vi "cm2nm_createGraphEnteredPoints.vi"(1 "EnteredPoints_in":T1[](array[typedef])) -> (0 "XY_graphOut":cluster{dbl[], dbl[]}[](array[cluster]))   [LabVIEW 2011]
doc: "Create a graph of the points in a data set by group number. There will be a separate line for each group number."
uses:
  cm2nm_coordinate_information_v2.ctl
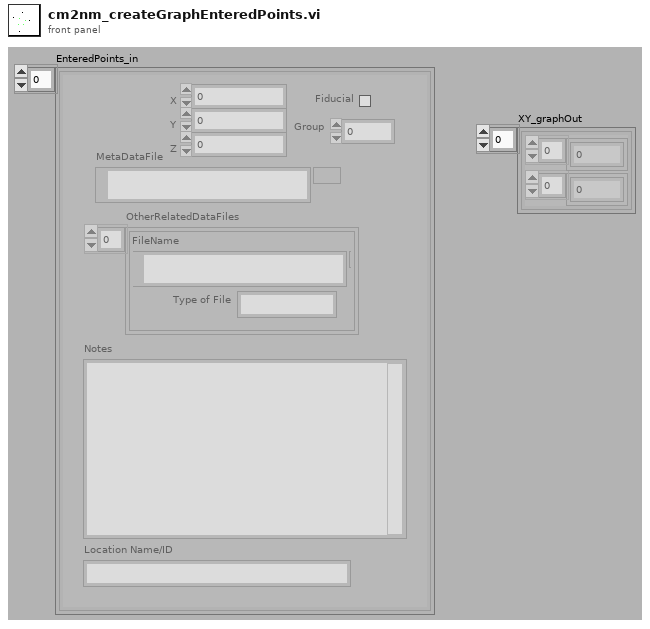
[diagram p1: front panel]
types:
  T1 = typedef "cm2nm_coordinate_information_v2.ctl" = cluster{"MetaDataFile":path, "X":dbl, "Y":dbl, "Z":dbl, "Group":i32, "Rotation":dbl[unit], "Fiducial":bool, "Magnification":dbl, "Working_Distance":dbl, "Notes":string, "Location Name/ID":string, "OtherRelatedDataFiles":cluster{"Type of File":string, "FileName":path}[], "Available":bool}
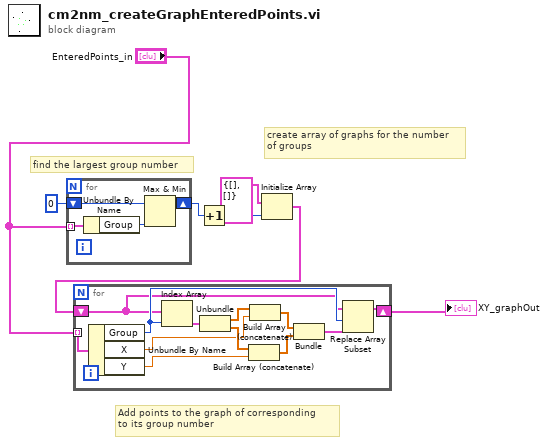
[diagram p0: block diagram]
diagram:
  # "Add points to the graph of corresponding\nto its group number"
  # "create array of graphs for the number\nof groups"
  # "find the largest group number"
  n1 = for {
    tunnel: "EnteredPoints_in" -> [w11] mode=indexing
    shift-right: [w9] -> w4
    shift-left: 0 -> [w8]
    n2 = Unbundle By Name(w11) -> ("Group"=w10:i32)
    n3 = Max & Min(x=w8, y=w10) -> (max(x,y)=w9:i32)  [unwired: 1 out]
  }
  n4 = Increment(x=w4) -> (x+1=w1:i32)
  n5 = Initialize Array(cluster{dbl[], dbl[]} {[], []}, w1) -> (w6:cluster{dbl[], dbl[]}[])
  n6 = for {
    tunnel: "EnteredPoints_in" -> [w23] mode=indexing
    shift-right: [w12] -> w7
    shift-left: w6 -> [w16]
    n7 = Unbundle By Name(w23) -> ("Group"=w17:i32, "X"=w18:dbl, "Y"=w19:dbl)
    n8 = Index Array(array=w16, index=w17) -> (element=w22:cluster{dbl[], dbl[]})
    n9 = Unbundle(w22) -> (w21:dbl[], w20:dbl[])
    n10 = Build Array (concatenate)(w20, w19) -> (w14:dbl[])
    n11 = Build Array (concatenate)(w21, w18) -> (w15:dbl[])
    n12 = Bundle(w15, w14) -> (w13:cluster{dbl[], dbl[]})  [unwired: 1 out]
    n13 = Replace Array Subset(array=w16, new element=w13, index=w17) -> (w12:cluster{dbl[], dbl[]}[])
  }
  "XY_graphOut" <- w7
